vi "Read t0.vi"(8 "error in (no error)":errorcluster, 11 "Const_WFM in":refnum<class "Const_WFM.lvclass">) -> (0 "error out":errorcluster, 2 "t0":timestamp, 3 "Const_WFM out":refnum<class "Const_WFM.lvclass">)   [LabVIEW 2021, in "Const_WFM.lvclass"]
uses:
  Const_WFM.lvclass
  Const_WFM.lvclass/Const_WFM.ctl
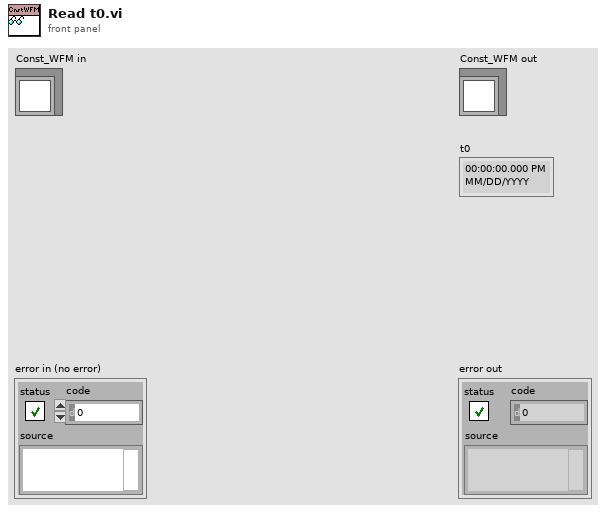
[diagram p1: front panel]
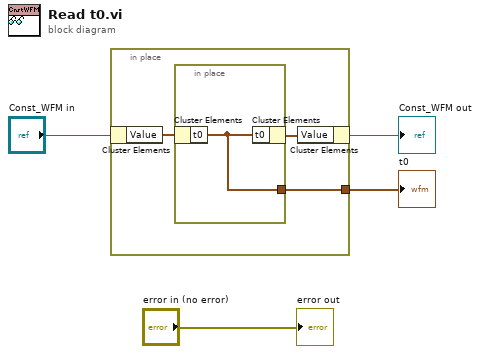
[diagram p0: block diagram]
diagram:
  n1 = in-place {
    in-place-border: [w5] -> w1
    n2 = in-place-cluster #1("Const_WFM in") -> ("Value"=w7:waveform(dbl))
    n3 = in-place {
      in-place-border: [w8] -> w5
      n4 = in-place-cluster #2(w7) -> ("t0"=w8:timestamp)
      n5 = in-place-cluster #2("t0"=w8) -> (w6:waveform(dbl))
    }
    n6 = in-place-cluster #1("Value"=w6) -> (→"Const_WFM out":refnum<class "Const_WFM.lvclass">)
  }
  "t0" <- w1
  "error out" <- "error in (no error)"
